vi "DataToClstr.vi"(8 "error in (no error)":errorcluster, 11 "CRDS Cell Data in":refnum<class "CRDS Cell Data.lvclass">) -> (0 "error out":errorcluster, 2 "DataOut":T3, 3 "CRDS Cell Data out":refnum<class "CRDS Cell Data.lvclass">)   [LabVIEW 2011, in "CRDS Cell Data.lvclass"]
uses:
  CRDS Cell Data.lvclass
  PAS_CRDS new/CRDS/Controls/extparam.ctl
  PAS_CRDS new/CRDS/Controls/calData.ctl
  CRDS Cell Data.lvclass/CRDS Cell Data.ctl
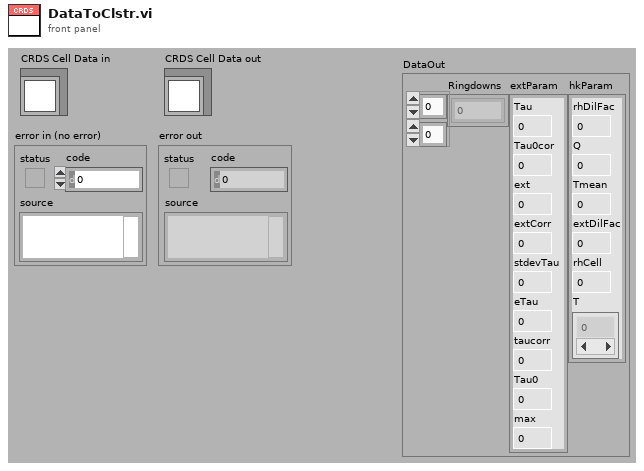
[diagram p1: front panel]
types:
  T1 = typedef "extparam.ctl" = cluster{"Tau":sgl, "Tau0cor":sgl, "ext":sgl, "extCorr":sgl, "stdevTau":sgl, "eTau":sgl, "taucorr":sgl, "Tau0":sgl, "max":sgl}
  T2 = typedef "calData.ctl" = cluster{"rhDilFac":sgl, "Q":sgl, "Tmean":sgl, "extDilFac":sgl, "rhCell":sgl, "T":sgl[]}
  T3 = cluster{"Ringdowns":i16[][], "extParam":T1, "hkParam":T2}
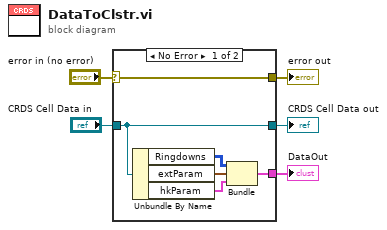
[diagram p0: block diagram]
diagram:
  n1 = case shown="No Error" "error in (no error)" {
    selector: "error in (no error)" -> [w11 w13]
    tunnel: [w11 w13] -> w4
    tunnel: [w10 w12] -> w2
    tunnel: "CRDS Cell Data in" -> [w10 w12]
    tunnel: [w6 _] -> w1
    frame No Error {
      n2 = Unbundle By Name(w10) -> ("Ringdowns"=w9:i16[][], "extParam"=w8:T1, "hkParam"=w7:T2)
      n3 = Bundle("Ringdowns"=w9, "extParam"=w8, "hkParam"=w7) -> (w6:T3)  [unwired: 1 in]
    }
    frame Error {
    }
  }
  "error out" <- w4
  "CRDS Cell Data out" <- w2
  "DataOut" <- w1
